vi "SendData_CANUSB.vi"(3 "error out 5":errorcluster, 4 "Msg":T1, 5 "VISA res_in":refnum<visa-resource-name>) -> (0 "error out 6":errorcluster, 1 "read buffer 2":string, 2 "status_1_OK":i32)   [LabVIEW 2017]
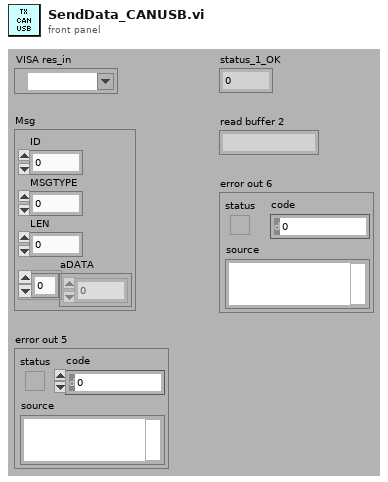
[diagram p1: front panel]
types:
  T1 = cluster{"ID":u32, "MSGTYPE":u8, "LEN":u8, "aDATA":u8[]}
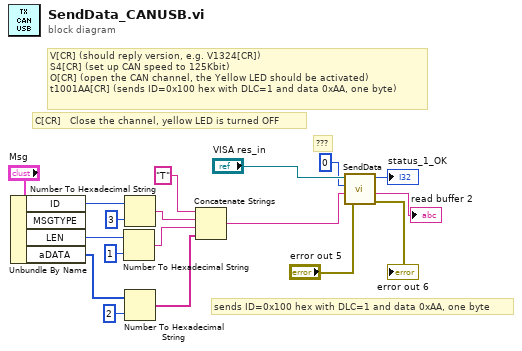
[diagram p0: block diagram]
diagram:
  # "???"
  # "C[CR]   Close the channel, yellow LED is turned OFF"
  # "sends ID=0x100 hex with DLC=1 and data 0xAA, one byte"
  # "V[CR] (should reply version, e.g. V1324[CR])\nS4[CR] (set up CAN speed to 125Kbit)\nO[CR] (open the CAN channel, the Yellow LED should be activated)\nt1001AA[CR] (sends ID=0x100 hex with DLC=1 and data 0xAA, one byte)"
  n1 = Unbundle By Name("Msg") -> ("ID"=w10:u32, "LEN"=w6:u8, "aDATA"=w4:u8[])  [unwired: 1 out]
  n2 = Number To Hexadecimal String(1:i16 1 ("width (-)"), 2:w6) -> (0:w5:string)
  n3 = Number To Hexadecimal String(1:i16 3 ("width (-)"), 2:w10) -> (0:w8:string)
  n4 = Number To Hexadecimal String(1:i16 2 ("width (-)"), 2:w4) -> (0:w2:string[])
  n5 = Concatenate Strings("T" ("String"), w8, w5, w2) -> (w1:string)
  n6 = call "SendData.vi"("error out 2"="error out 5", "String"=w1, "byte count"=u32 0, "VISA resource name out 2"="VISA res_in") -> ("error out"=→"error out 6":errorcluster, "read buffer"=→"read buffer 2":string, "status_1_OK"=→"status_1_OK":i32)  [unwired: 1 out]
